vi "oa_Calculate Delay of CIC Decimation Interpolation Filter.vi"(8 "lp filter settings":T1={"coefficients"=[], "factor"=1} {"coefficients" format="%.2f"}, 9 "compensation filter settings":T1={"coefficients"=[], "factor"=1} {"coefficients" format="%.2f"}, 10 "CIC decimation setting":T2) -> (3 "delay":i32)   [LabVIEW 2017, in "SoundVib_Resampling.lvlib"]
uses:
  <vilib>/addons/Sound and Vibration/Order Analysis/Resample Order Tracking/SoundVib_Resampling.lvlib
  <vilib>/addons/_NISVFA/_Shared subVIs/Controls/OAT Decimation Filter.ctl
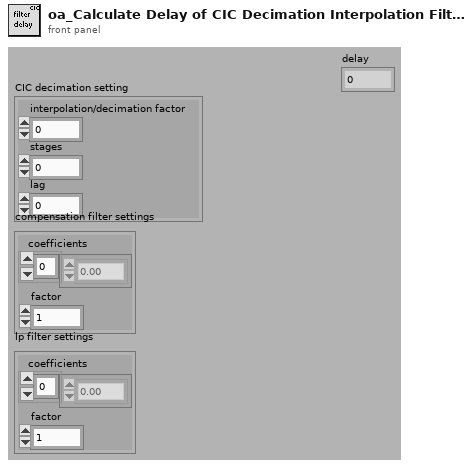
[diagram p1: front panel]
types:
  T1 = typedef "OAT Decimation Filter.ctl" = cluster{"coefficients":dbl[], "factor":i32}
  T2 = cluster{"interpolation/decimation factor":i32, "stages":i32, "lag":i32}
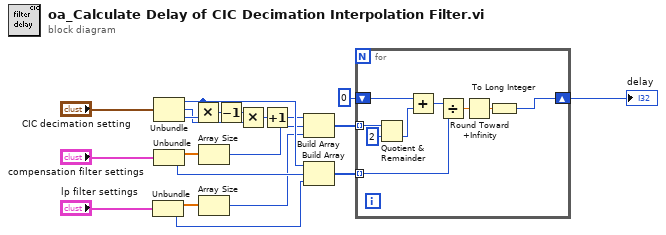
[diagram p0: block diagram]
diagram:
  n1 = Unbundle("lp filter settings") -> ("coefficients"=w11:dbl[], "factor"=w9:i32)
  n2 = Unbundle("CIC decimation setting") -> ("interpolation/decimation factor"=w8:i32, "stages"=w13:i32, "lag"=w14:i32)
  n3 = Unbundle("compensation filter settings") -> ("coefficients"=w12:dbl[], "factor"=w10:i32)
  n4 = Multiply(x=w8, y=w14) -> (x*y=w17:i32)
  n5 = Array Size(array=w12) -> (size(s)=w4:i32)
  n6 = Array Size(array=w11) -> (size(s)=w3:i32)
  n7 = Decrement(x=w17) -> (x-1=w16:i32)
  n8 = Multiply(x=w16, y=w13) -> (x*y=w15:i32)
  n9 = Increment(x=w15) -> (x+1=w5:i32)
  n10 = Build Array(w5, w4, w3) -> (w2:i32[])
  n11 = Build Array(w8, w10, w9) -> (w6:i32[])
  n12 = for {
    tunnel: w6 -> [w27] mode=indexing
    shift-right: [w26] -> w7
    shift-left: 0 -> [w22]
    tunnel: w2 -> [w24] mode=indexing
    n13 = Quotient & Remainder(x=w24, y=2) -> (floor(x/y)=w23:i32)  [unwired: 1 out]
    n14 = Add(x=w22, y=w23) -> (x+y=w21:i32)
    n15 = Divide(x=w21, y=w27) -> (x/y=w28:dbl)
    n16 = Round Toward +Infinity(x=w28) -> (ceil(x): smallest int >= x=w29:dbl)
    n17 = To Long Integer(number=w29) -> (32bit integer=w26:i32)
  }
  "delay" <- w7
